vi "test_fb_pid.vi"() -> ()   [LabVIEW 2016]
uses:
  <vilib>/rvi/DesktopExecutionNode/Execution/niFpgaDEN_Execute.vi
  <vilib>/rvi/DesktopExecutionNode/DesktopExecutionNode.xnode
panel:
  in  "pidEnableTime":i32=200
  out "zHeight":cluster{i32[], dbl[]}(graph)
  in  "offsetSwitchTime":i32
  in  "offset2":dbl
  in  "offset1":dbl
  out "output":T1(array[cluster])
  in  "fbParams":T2={"enable"=TRUE, "setPoint"=0.0, "pGain"=0.001007080078125, "iGain"=0.00099945068359375, "gainScale"=0}
  in  "liftOffParams":T3={"liftHeight"=0.0, "disengagePos"=-1.0, "liftOff"=FALSE}
  in  "manualMotion":T4
  in  "limits":T5
  in  "sampleValidDec":i32=3
  in  "cycleLength":i32
  in  "inputNoiseScale":dbl=500.0
  out "inEndOfCycle":bool[](array[boolean])
  out "dataIn":dbl[](graph)
  in  "numTicks":i32=600
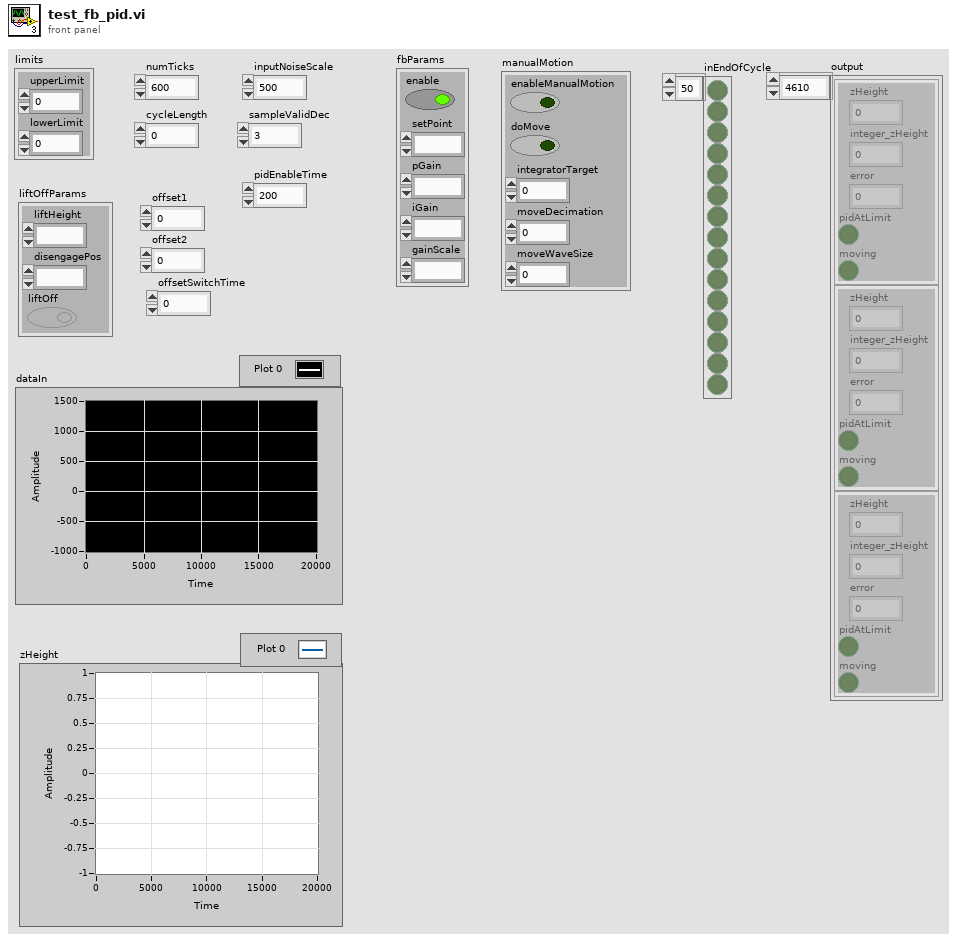
[diagram p1: front panel]
types:
  T1 = cluster{"zHeight":fxp<+/-,28,1>, "integer_zHeight":i16, "error":fxp<+/-,25,2>, "pidAtLimit":bool, "moving":bool}[]
  T2 = cluster{"enable":bool, "setPoint":fxp<+/-,17,1>, "pGain":fxp<+/-,20,4>, "iGain":fxp<+/-,20,1>, "gainScale":i8}
  T3 = cluster{"liftHeight":fxp<+/-,15,4>, "disengagePos":fxp<+/-,22,1>, "liftOff":bool}
  T4 = cluster{"enableManualMotion":bool, "doMove":bool, "integratorTarget":fxp<+/-,22,2>, "moveDecimation":u16, "moveWaveSize":u16}
  T5 = cluster{"upperLimit":fxp<+/-,28,4>, "lowerLimit":fxp<+/-,28,4>}
  T6 = cluster{"zHeight":fxp<+/-,28,1>, "integer_zHeight":i16, "error":fxp<+/-,25,2>, "pidAtLimit":bool, "moving":bool}
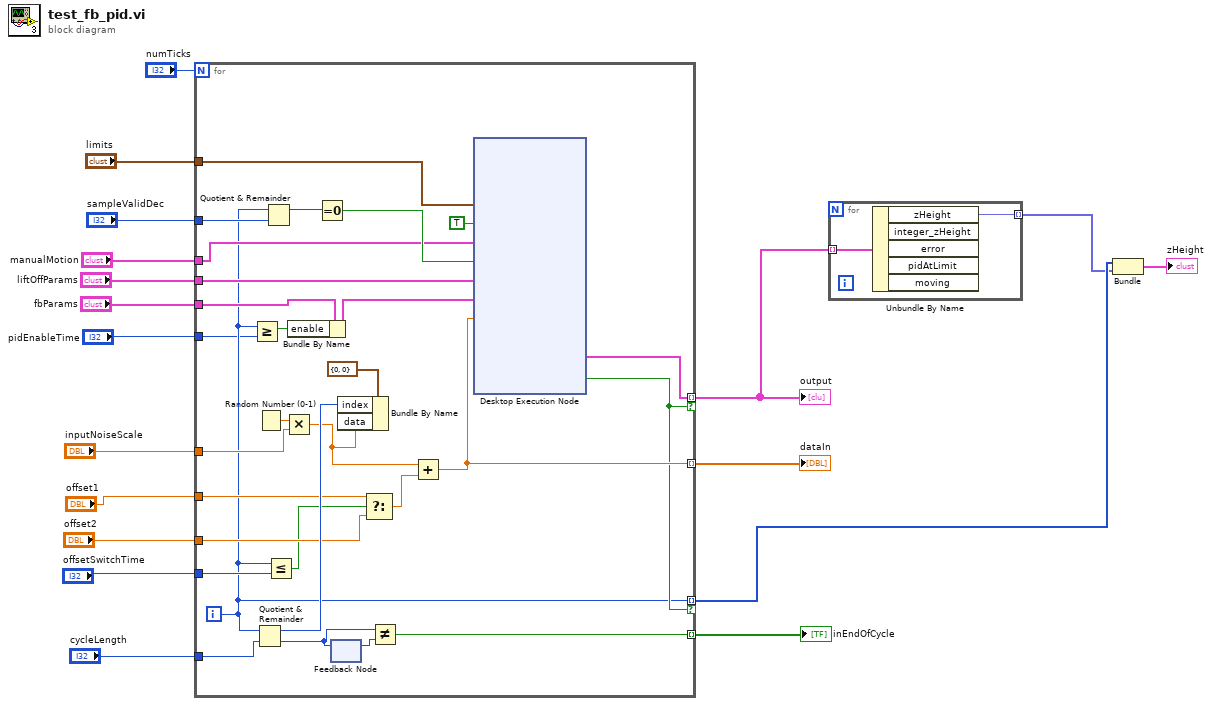
[diagram p0: block diagram]
diagram:
  n1 = for {
    N: "numTicks" -> [_]
    tunnel: [w25] -> w17 mode=indexing
    tunnel: [w42] -> w16 mode=indexing
    tunnel: "inputNoiseScale" -> [w41]
    tunnel: "cycleLength" -> [w40]
    tunnel: "sampleValidDec" -> [w39]
    tunnel: "limits" -> [w37]
    tunnel: "manualMotion" -> [w34]
    tunnel: "liftOffParams" -> [w33]
    tunnel: "fbParams" -> [w32]
    tunnel: [w30] -> w5 mode=indexing if=w23
    tunnel: "offset1" -> [w29]
    tunnel: "offset2" -> [w28]
    tunnel: "offsetSwitchTime" -> [w27]
    tunnel: [w20] -> w3 mode=indexing if=w23
    tunnel: "pidEnableTime" -> [w19]
    i -> [w20]
    n2 = Greater Or Equal?(x=w20, y=w19) -> (x >= y?=w21:bool)
    n3 = Quotient & Remainder(x=w20, y=w40) -> (x-y*floor(x/y)=w44:i32, floor(x/y)=w43:i32)
    n4 = Random Number (0-1)() -> (number: 0 to 1=w46:dbl)
    n5 = Quotient & Remainder(x=w20, y=w39) -> (x-y*floor(x/y)=w38:i32)  [unwired: 1 out]
    n6 = Less Or Equal?(x=w20, y=w27) -> (x <= y?=w26:bool)
    n7 = Multiply(x=w46, y=w41) -> (x*y=w31:dbl)
    n8 = Bundle By Name(cluster=w32, "enable"=w21) -> (w22:T2)
    n9 = Equal To 0?(x=w38) -> (x = 0?=w36:bool)
    n10 = feedback-in #1(w43) -> ()
    n11 = feedback #1() -> (w45:i32)  [unwired: 1 in]
    n12 = Bundle By Name(cluster=cluster{"index":u16, "data":i16} {"index"=0, "data"=0} ("input"), "index"=w44, "data"=w31) -> ()  [unwired: 1 out]
    n13 = Select(t=w29, s=w26, f=w28) -> (s? t:f=w24:dbl)
    n14 = Not Equal?(x=w43, y=w45) -> (x != y?=w42:bool)
    n15 = Add(x=w31, y=w24) -> (x+y=w25:dbl)
    n16 = xnode "Desktop Execution Node"("limits"=w37, "ready for output (T)"=TRUE, "manualMotion"=w34, "input valid"=w36, "liftOffParams"=w33, "fbParams"=w22, "input"=w25) -> ("output valid"=w23:bool, "output"=w30:T6)  [unwired: 1 in, 2 out]
  }
  "dataIn" <- w17
  "inEndOfCycle" <- w16
  "output" <- w5
  n17 = for {
    tunnel: w5 -> [w49] mode=indexing
    tunnel: [w48] -> w2 mode=indexing
    n18 = Unbundle By Name(w49) -> ("zHeight"=w48:fxp<+/-,28,1>)  [unwired: 4 out]
  }
  n19 = Bundle(w3, w2) -> (→"zHeight":cluster{i32[], fxp<+/-,28,1>[]})  [unwired: 1 in]
